vi "Get Library.vi"(7 "error if not found":bool=TRUE, 8 "error in (no error)":errorcluster, 10 "library name":string, 11 "project in":refnum<vi>) -> (0 "error out":errorcluster, 1 "found":bool, 2 "library item":refnum<vi>, 3 "project out":refnum<vi>)   [LabVIEW 2021, in "MeasurementService Editor.lvlib"]
uses:
  MeasurementService Editor.lvlib
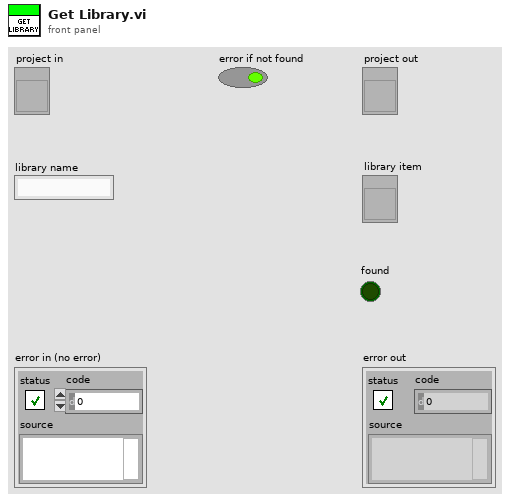
[diagram p1: front panel]
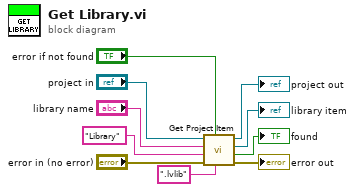
[diagram p0: block diagram]
diagram:
  n1 = call "Get Project Item.vi"("library file extension"=".lvlib", "error if not found"="error if not found", "error in (no error)"="error in (no error)", "library type"="Library", "library name"="library name", "project in"="project in") -> ("error out"=→"error out":errorcluster, "found"=→"found":bool, "library item"=→"library item":refnum<vi>, "project out"=→"project out":refnum<vi>)  [unwired: 2 in]
